vi "Step SSS.vi"(11 "Step Actuator Values In":T1) -> (3 "Step Actuator Values Out":T1)   [LabVIEW 2014]
uses:
  Step Deployment Actuator Values.ctl
  <vilib>/Rock Robotics/WPI/Solenoid/WPI_SolenoidValue.ctl
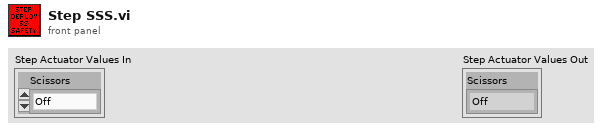
[diagram p1: front panel]
types:
  T1 = typedef "Step Deployment Actuator Values.ctl" = cluster{"Scissors":T2}
  T2 = typedef "WPI_SolenoidValue.ctl" = enum16{"Off", "On", "Forward", "Reverse"}
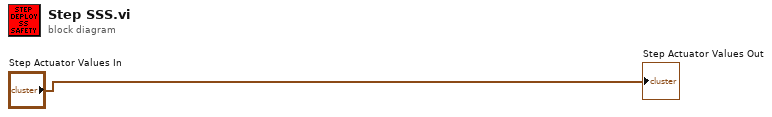
[diagram p0: block diagram]
diagram:
  "Step Actuator Values Out" <- "Step Actuator Values In"
